vi "弯曲双线性曲线图.vi"(0 "文件路径输入控件":path) -> (1 "弯曲刚度值 2":dbl, 2 "弯曲刚度值1":dbl, 3 "XY Graph":cluster{"Y":dbl[], "Y":dbl[]}[](graph) caption="弯曲刚度")   [LabVIEW 2016]
uses:
  <vilib>/Analysis/NI_AALPro.lvlib
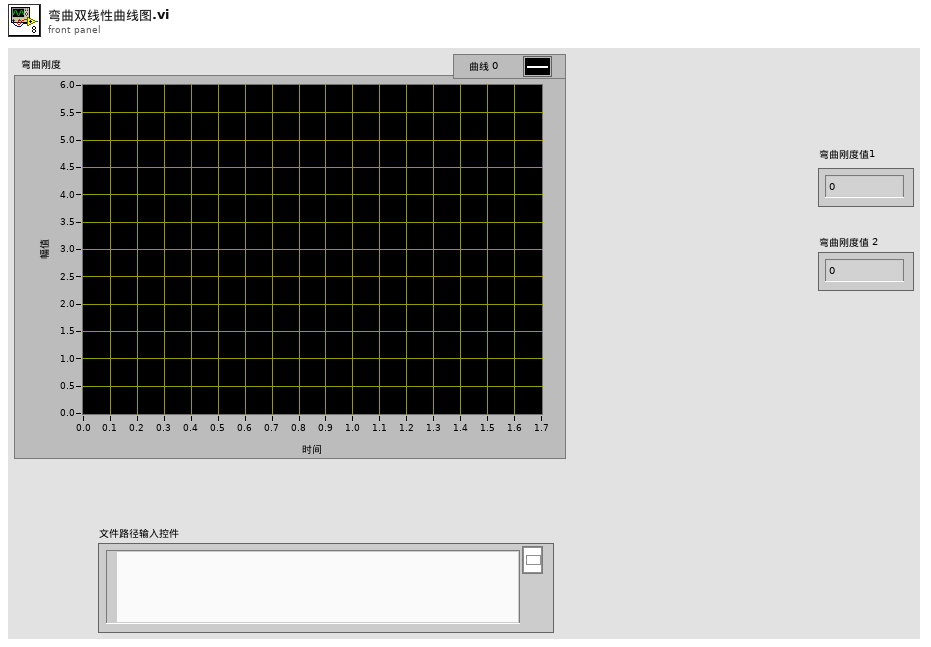
[diagram p1: front panel]
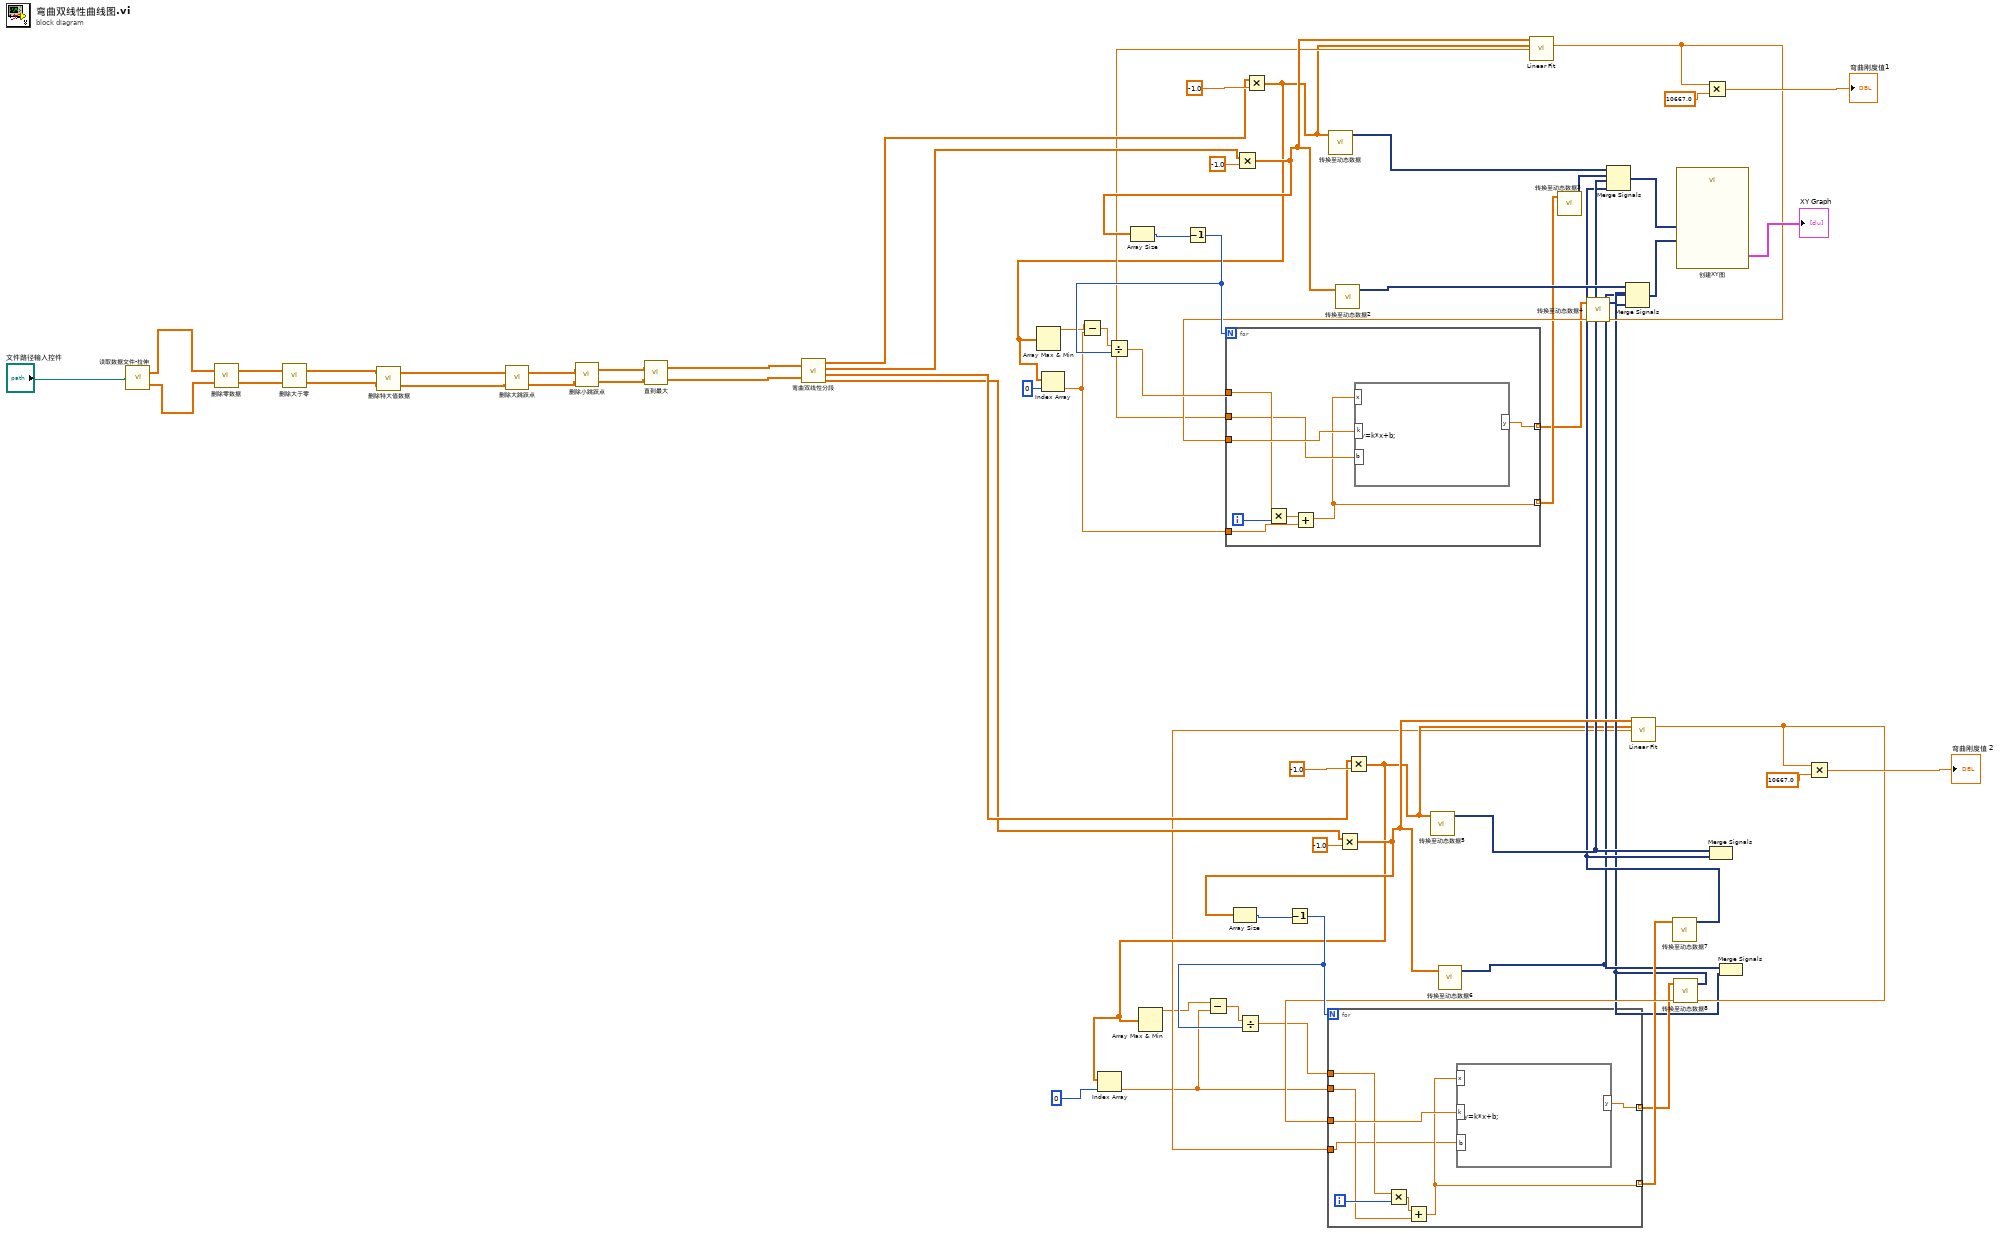
[diagram p0: block diagram]
diagram:
  n1 = call "读取数据文件-拉伸.vi"("文件路径（使用对话框）"="文件路径输入控件") -> ("第一列"=w63:dbl[], "第二列"=w62:dbl[])
  n2 = call "删除零数据.vi"("数组－数值 2"=w62, "数组－数值"=w63) -> ("第二列"=w60:dbl[], "第一列"=w61:dbl[])
  n3 = call "删除大于零.vi"("数组－数值 2"=w60, "数组－数值"=w61) -> ("第二列"=w54:dbl[], "第一列"=w55:dbl[])
  n4 = call "删除特大值数据.vi"("数组－数值 2"=w54, "数组－数值"=w55) -> ("数组 6"=w52:dbl[], "数组 5"=w53:dbl[])
  n5 = call "删除大跳跃点.vi"("数组－数值 2"=w52, "数组－数值"=w53) -> ("数组 6"=w58:dbl[], "数组 5"=w59:dbl[])
  n6 = call "删除小跳跃点.vi"("数组－数值 2"=w58, "数组－数值"=w59) -> ("第二列"=w56:dbl[], "第一列"=w57:dbl[])
  n7 = call "直到最大.vi"("数组－数值 2"=w56, "数组－数值"=w57) -> ("子数组 2"=w50:dbl[], "子数组"=w51:dbl[])
  n8 = call "弯曲双线性分段.vi"("数组－数值"=w51, "数组－数值 2"=w50) -> ("子数组"=w31:dbl[], "子数组 2"=w30:dbl[], "子数组 3"=w19:dbl[], "子数组 4"=w18:dbl[])
  n9 = Multiply(x=w30, y=-1.0) -> (x*y=w34:dbl[])
  n10 = Array Size(array=w34) -> (size(s)=w44:i32)
  n11 = Decrement(x=w44) -> (x-1=w43:i32)
  n12 = Multiply(x=w31, y=-1.0) -> (x*y=w4:dbl[])
  n13 = Array Max & Min(array=w4) -> (max value=w2:dbl)  [unwired: 3 out]
  n14 = Index Array(array=w4, index=0 ("索引")) -> (element=w1:dbl)
  n15 = Subtract(x=w2, y=w1) -> (x-y=w3:dbl)
  n16 = Divide(x=w3, y=w43) -> (x/y=w42:dbl)
  n17 = call "转换至动态数据"("Array"=w4) -> ("Dynamic Data Type"=w49:dynamicdata)  [unwired: 3 in]
  n18 = call "转换至动态数据2"("Array"=w34) -> ("Dynamic Data Type"=w48:dynamicdata)  [unwired: 3 in]
  n19 = Multiply(x=w18, y=-1.0) -> (x*y=w22:dbl[])
  n20 = Array Size(array=w22) -> (size(s)=w29:i32)
  n21 = Decrement(x=w29) -> (x-1=w28:i32)
  n22 = Multiply(x=w19, y=-1.0) -> (x*y=w13:dbl[])
  n23 = Index Array(array=w13, index=0 ("索引")) -> (element=w7:dbl)
  n24 = Array Max & Min(array=w13) -> (max value=w8:dbl)  [unwired: 3 out]
  n25 = Subtract(x=w8, y=w7) -> (x-y=w9:dbl)
  n26 = Divide(x=w9, y=w28) -> (x/y=w11:dbl)
  n27 = call "转换至动态数据5"("Array"=w13) -> ("Dynamic Data Type"=w17:dynamicdata)  [unwired: 3 in]
  n28 = call "转换至动态数据6"("Array"=w22) -> ("Dynamic Data Type"=w15:dynamicdata)  [unwired: 3 in]
  n29 = call <vilib>:"Linear Fit.vi"("Y"=w34, "X"=w4) -> ("slope"=w35:dbl, "intercept"=w6:dbl)  [unwired: 9 in, 3 out]
  n30 = for {
    N: w43 -> [_]
    tunnel: w35 -> [w72]
    tunnel: [w71] -> w32 mode=indexing
    tunnel: [w66] -> w33 mode=indexing
    tunnel: w42 -> [w70]
    tunnel: w6 -> [w68]
    tunnel: w1 -> [w65]
    i -> [w69]
    n31 = Multiply(x=w70, y=w69) -> (x*y=w67:dbl)
    n32 = Add(x=w67, y=w65) -> (x+y=w66:dbl)
    n33 = formula code="y=k*x+b;"("x"=w66, "k"=w72, "b"=w68) -> ("y"=w71:dbl)
  }
  n34 = call "转换至动态数据3"("Array"=w33) -> ("Dynamic Data Type"=w41:dynamicdata)  [unwired: 3 in]
  n35 = call "转换至动态数据4"("Array"=w32) -> ("Dynamic Data Type"=w40:dynamicdata)  [unwired: 3 in]
  n36 = call <vilib>:"Linear Fit.vi"("Y"=w22, "X"=w13) -> ("slope"=w23:dbl, "intercept"=w10:dbl)  [unwired: 9 in, 3 out]
  n37 = for {
    N: w28 -> [_]
    tunnel: w23 -> [w80]
    tunnel: [w79] -> w20 mode=indexing
    tunnel: [w74] -> w21 mode=indexing
    tunnel: w11 -> [w78]
    tunnel: w7 -> [w76]
    tunnel: w10 -> [w73]
    i -> [w77]
    n38 = Multiply(x=w78, y=w77) -> (x*y=w75:dbl)
    n39 = Add(x=w75, y=w76) -> (x+y=w74:dbl)
    n40 = formula code="y=k*x+b;"("x"=w74, "k"=w80, "b"=w73) -> ("y"=w79:dbl)
  }
  n41 = call "转换至动态数据7"("Array"=w21) -> ("Dynamic Data Type"=w16:dynamicdata)  [unwired: 3 in]
  n42 = Merge Signals(w49, w41, w17, w16) -> (w47:dynamicdata)
  n43 = call "转换至动态数据8"("Array"=w20) -> ("Dynamic Data Type"=w14:dynamicdata)  [unwired: 3 in]
  n44 = Merge Signals(w48, w40, w15, w14) -> (w46:dynamicdata)
  n45 = call "创建XY图"("Y Input"=w46, "X Input"=w47) -> ("XY Graph"=→"XY Graph":cluster{"X":dbl[], "Y":dbl[]}[])  [unwired: 8 in, 1 out]
  n46 = Multiply(x=w35, y=10667.0) -> (x*y=→"弯曲刚度值1":dbl)
  n47 = Merge Signals(w17, w16) -> ()  [unwired: 1 out]
  n48 = Merge Signals(w15, w14) -> ()  [unwired: 1 out]
  n49 = Multiply(x=w23, y=10667.0) -> (x*y=→"弯曲刚度值 2":dbl)
